vi "Print Control.vi"(8 "error in (no error)":errorcluster, 10 "Start":bool, 11 "Main.lvlib:Main.lvclass":refnum<class "Main.lvclass">) -> (0 "error out":errorcluster, 3 "Actor out":refnum<class "Actor.lvclass">)   [LabVIEW 2018, in "Main.lvlib" / "Main.lvclass"]
uses:
  Main.lvclass
  C:/Program Files/National Instruments/LabVIEW 2018/vi.lib/ActorFramework/Actor/Actor.lvclass
  <vilib>/ActorFramework/Actor/Actor.lvclass
  Main.lvclass/Main.ctl
  Feeder Actor/Feeder Messages/Print Reset Msg/Print Reset Msg.lvclass
  MFC Actor/MFC Messages/Set Print Msg/Set Print Msg.lvclass
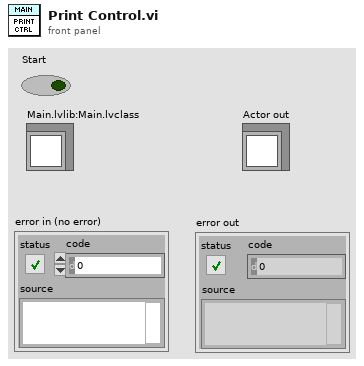
[diagram p1: front panel]
types:
  T1 = enum8{"Enabled", "Disabled", "Disabled and Grayed Out"}
  T2 = cluster{"Chamber Pressure":refnum<vi>, "Stage Sub Panel":refnum<vi>, "Feeder Pressure":refnum<vi>, "Inner MFC Sub Panel":refnum<vi>, "Outer MFC Sub Panel":refnum<vi>, "Feeder Sub Panel":refnum<vi>}
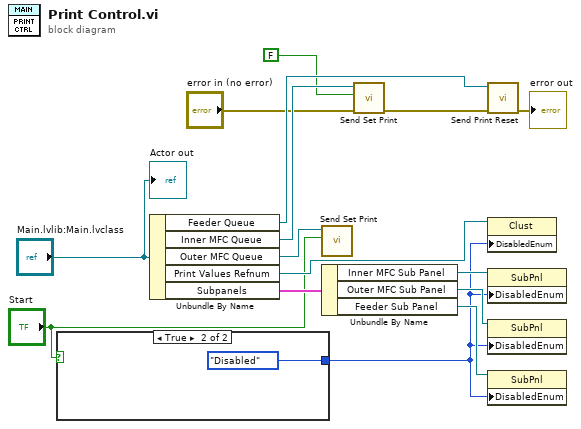
[diagram p0: block diagram]
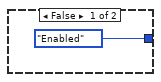
[diagram p2: hidden frame]
diagram:
  n1 = case shown="True" "Start" {
    tunnel: [T1."Enabled" ("Disabled") T1."Disabled" ("Disabled")] -> w2
    frame False {
    }
    frame True {
    }
  }
  n2 = Unbundle By Name("Main.lvlib:Main.lvclass") -> ("Feeder Queue"=w9:refnum<class "Message Enqueuer.lvclass">, "Inner MFC Queue"=w7:refnum<class "Message Enqueuer.lvclass">, "Outer MFC Queue"=w6:refnum<class "Message Enqueuer.lvclass">, "Print Values Refnum"=w14:refnum<vi>, "Subpanels"=w10:T2)
  n3 = call "Send Set Print.vi"("On?"="Start", "Message Enqueuer in"=w6) -> ()  [unwired: 8 in, 2 out]
  n4 = Unbundle By Name(w10) -> ("Inner MFC Sub Panel"=w13:refnum<vi>, "Outer MFC Sub Panel"=w12:refnum<vi>, "Feeder Sub Panel"=w11:refnum<vi>)
  n5 = call "Send Set Print.vi"("error in (no error)"="error in (no error)", "On?"=FALSE, "Message Enqueuer in"=w7) -> ("error out"=w8:errorcluster)  [unwired: 7 in, 1 out]
  n6 = call "Send Print Reset.vi"("error in (no error)"=w8, "Message Enqueuer in"=w9) -> ("error out"=→"error out":errorcluster)  [unwired: 8 in, 1 out]
  n7 = property class="Clust"(reference=w14, "DisabledEnum"=w2) -> ()  [unwired: 1 in, 2 out]
  n8 = property class="SubPnl"(reference=w13, "DisabledEnum"=w2) -> ()  [unwired: 1 in, 2 out]
  n9 = property class="SubPnl"(reference=w12, "DisabledEnum"=w2) -> ()  [unwired: 1 in, 2 out]
  n10 = property class="SubPnl"(reference=w11, "DisabledEnum"=w2) -> ()  [unwired: 1 in, 2 out]
  "Actor out" <- "Main.lvlib:Main.lvclass"
